vi "read_ini_SavedPos.vi"(8 "error in (no error)":errorcluster caption="错误输入（无错误）", 10 "file ref in":T1, 11 "MotorSystem 输入":refnum<class "MotorSystem.lvclass">) -> (0 "error out":errorcluster caption="错误输出", 2 "file ref out":T1, 3 "MotorSystem 输出":refnum<class "MotorSystem.lvclass">)   [LabVIEW 2016, in "MotionControl_UFO_3DOF.lvlib" / "MotorSystem.lvclass"]
uses:
  <userlib>/MotionControl_UFO_3DOF/MotorSystem/MotorSystem.lvclass
  <vilib>/Utility/config.llb/Config Data RefNum.ctl
  <userlib>/MotionControl_UFO_3DOF/MotorSystem/SavedPosCluster.ctl
  <userlib>/MotionControl_UFO_3DOF/MotorSystem/CommandList.ctl
  <userlib>/MotionControl_UFO_3DOF/MotorSystem/cmd_system.ctl
  <userlib>/MotionControl_UFO_3DOF/MotorSystem/SavedDimensionCluster.ctl
  <userlib>/MotionControl_UFO_3DOF/OneMotion/unit mode.ctl
  <userlib>/MotionControl_UFO_3DOF/MotorSystem/MotorSystem.lvclass/MotorSystem.ctl
  <vilib>/Utility/config.llb/Read Key (I32).vi
  <vilib>/Utility/config.llb/Read Key (String).vi
  <vilib>/Utility/config.llb/Read Key (Double).vi
  <vilib>/Utility/config.llb/NI_LVConfig.lvlib
  <userlib>/MotionControl_UFO_3DOF/OneMotion/OneMotion.lvclass
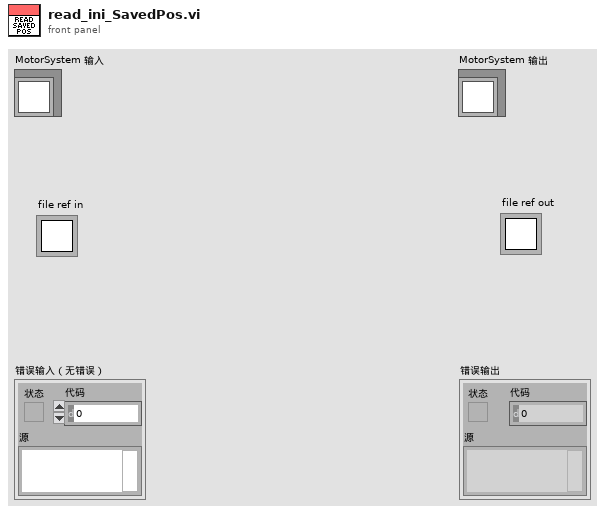
[diagram p1: front panel]
types:
  T1 = typedef "NI_LVConfig.lvlib/Config Data RefNum.ctl" = refnum<k1>
  T2 = typedef "MotionControl_UFO_3DOF.lvlib/MotorSystem.lvclass/SavedPosCluster.ctl" = cluster{"name":string, "command list":T3}
  T3 = typedef "MotionControl_UFO_3DOF.lvlib/MotorSystem.lvclass/CommandList.ctl" = cluster{"cmd":T4, "cmd info":T5[]}[]
  T4 = typedef "MotionControl_UFO_3DOF.lvlib/MotorSystem.lvclass/cmd_system.ctl" = enum16{"NONE", "MOVE_SYSTEM", "WAIT_UNTIL_MOVE_DONE", "EXIT", "WAIT_UNTIL_SELECTED_MOVE_DONE", "WAIT_A_TIME"}
  T5 = typedef "MotionControl_UFO_3DOF.lvlib/MotorSystem.lvclass/SavedDimensionCluster.ctl" = cluster{"dimension name":string, "pos":dbl, "unit mode":T6, "unit conversion ratio":dbl}
  T6 = typedef "MotionControl_UFO_3DOF.lvlib/OneMotion.lvclass/unit mode.ctl" = enum16{"motor (pulse)", "linear (mm) or radial (degree)"}
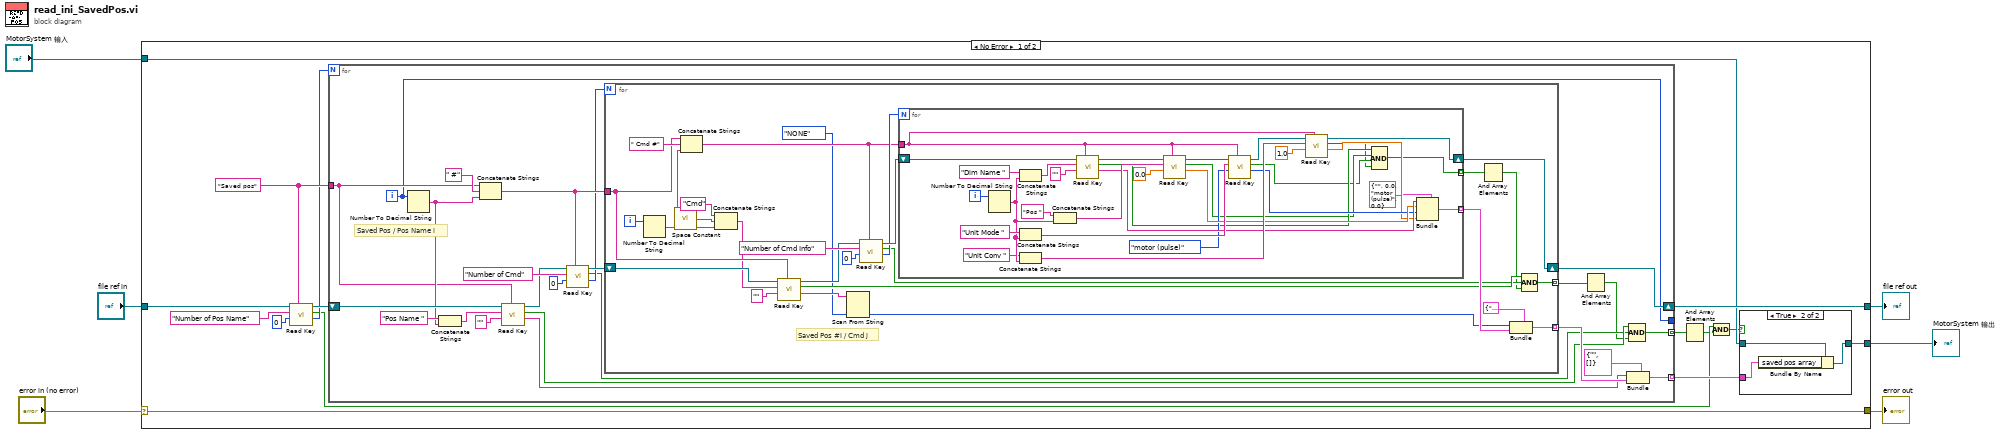
[diagram p0: block diagram]
diagram:
  n1 = case shown="No Error" "error in (no error)" {
    selector: "error in (no error)" -> [w21 w110]
    tunnel: [w21 w110] -> w5
    tunnel: [w11 w109] -> w3
    tunnel: "MotorSystem 输入" -> [w12 w109]
    tunnel: "file ref in" -> [w17 w108]
    tunnel: [w20 w108] -> w1
    frame No Error {
      w18 = "Saved pos"
      n2 = call-poly <vilib>:"Read Key.vi"("section"=w18, "default value"=0, "key"="Number of Pos Name", "refnum"=w17) -> ("value"=w14:i32, "found?"=w9:bool, "refnum out"=w16:T1)  [unwired: 4 in, 1 out]
      n3 = for {
        N: w14 -> [_]
        shift-right: [w46] -> w20
        shift-left: w16 -> [w47]
        tunnel: w18 -> [w43]
        tunnel: [w33] -> w13 mode=indexing
        tunnel: [w41] -> _
        tunnel: [w26] -> w10 mode=indexing
        i -> [w41]
        # "Saved Pos / Pos Name i"
        n4 = Number To Decimal String(number=w41) -> (decimal integer string=w44:string)  [unwired: 1 in]
        n5 = Concatenate Strings("Pos Name ", w44) -> (w48:string)
        n6 = Concatenate Strings(w43, " #", w44) -> (w39:string)
        n7 = call-poly <vilib>:"Read Key.vi"("section"=w43, "default value"="", "key"=w48, "refnum"=w47) -> ("value"=w34:string, "found?"=w29:bool, "refnum out"=w31:T1)  [unwired: 4 in, 1 out]
        n8 = call-poly <vilib>:"Read Key.vi"("section"=w39, "default value"=0, "key"="Number of Cmd", "refnum"=w31) -> ("value"=w36:i32, "found?"=w28:bool, "refnum out"=w38:T1)  [unwired: 4 in, 1 out]
        n9 = for {
          N: w36 -> [_]
          tunnel: w39 -> [w69]
          tunnel: [w61] -> w35 mode=indexing
          shift-right: [w76] -> w46
          shift-left: w38 -> [w73]
          tunnel: [w54] -> w30 mode=indexing
          i -> [w70]
          # "Saved Pos #i / Cmd j"
          n10 = Number To Decimal String(number=w70) -> (decimal integer string=w72:string)  [unwired: 1 in]
          n11 = call <vilib>:"Space Constant.vi"() -> ("String"=w68:string)
          n12 = Concatenate Strings(w69, " Cmd #", w72) -> (w63:string)
          n13 = Concatenate Strings("Cmd", w68, w72) -> (w67:string)
          n14 = call-poly <vilib>:"Read Key.vi"("section"=w69, "default value"="", "key"=w67, "refnum"=w73) -> ("value"=w53:string, "found?"=w57:bool, "refnum out"=w58:T1)  [unwired: 4 in, 1 out]
          n15 = Scan From String(input string=w53, default 1=cmd_system."NONE" ("cmd")) -> (output 1=w50:T4)  [unwired: 3 in, 3 out]
          n16 = call-poly <vilib>:"Read Key.vi"("section"=w63, "default value"=0, "key"="Number of Cmd Info", "refnum"=w58) -> ("value"=w64:i32, "found?"=w56:bool, "refnum out"=w65:T1)  [unwired: 4 in, 1 out]
          n17 = for {
            N: w64 -> [_]
            shift-right: [w95] -> w76
            shift-left: w65 -> [w106]
            tunnel: w63 -> [w94]
            tunnel: [w85] -> w62 mode=indexing
            tunnel: [w77] -> w59 mode=indexing
            i -> [w84]
            n18 = Number To Decimal String(number=w84) -> (decimal integer string=w101:string)  [unwired: 1 in]
            n19 = Concatenate Strings("Dim Name ", w101) -> (w93:string)
            n20 = Concatenate Strings("Unit Mode ", w101) -> (w98:string)
            n21 = Concatenate Strings("Unit Conv ", w101) -> (w99:string)
            n22 = Concatenate Strings("Pos ", w101) -> (w104:string)
            n23 = call-poly <vilib>:"Read Key.vi"("section"=w94, "default value"="", "key"=w93, "refnum"=w106) -> ("value"=w91:string, "found?"=w81:bool, "refnum out"=w103:T1)  [unwired: 4 in, 1 out]
            n24 = call-poly <vilib>:"Read Key.vi"("section"=w94, "default value"=0.0, "key"=w104, "refnum"=w103) -> ("value"=w89:dbl, "found?"=w80:bool, "refnum out"=w97:T1)  [unwired: 4 in, 1 out]
            n25 = call-poly <vilib>:"Read Key.vi"("section"=w94, "default value"=unit_mode."motor (pulse)" ("unit mode"), "key"=w98, "refnum"=w97) -> ("value"=w87:i32, "found?"=w79:bool, "refnum out"=w96:T1)  [unwired: 4 in, 1 out]
            n26 = call-poly <vilib>:"Read Key.vi"("section"=w94, "default value"=1.0, "key"=w99, "refnum"=w96) -> ("value"=w86:dbl, "found?"=w78:bool, "refnum out"=w95:T1)  [unwired: 4 in, 1 out]
            n27 = Compound Arithmetic op=AND(w81, w80, w79, w78) -> (w77:bool)
            n28 = Bundle(cluster=T5 {"dimension name"="", "pos"=0.0, "unit mode"=enum."motor (pulse)", "unit conversion ratio"=0.0} ("a dimension cluster"), "dimension name"=w91, "pos"=w89, "unit mode"=w87, "unit conversion ratio"=w86) -> (w85:T5)
          }
          n29 = And Array Elements(Boolean array=w59) -> (logical AND=w55:bool)
          n30 = Bundle(cluster=cluster{"cmd":T4, "cmd info":T5[]} {"cmd"=enum."NONE", "cmd info"=[]} ("a saved pos"), "cmd"=w50, "cmd info"=w62) -> (w61:cluster{"cmd":T4, "cmd info":T5[]})
          n31 = Compound Arithmetic op=AND(w57, w56, w55) -> (w54:bool)
        }
        n32 = And Array Elements(Boolean array=w30) -> (logical AND=w27:bool)
        n33 = Bundle(cluster=T2 {"name"="", "command list"=[]} ("a saved pos cluster"), "name"=w34, "command list"=w35) -> (w33:T2)
        n34 = Compound Arithmetic op=AND(w29, w28, w27) -> (w26:bool)
      }
      n35 = And Array Elements(Boolean array=w10) -> (logical AND=w8:bool)
      n36 = Compound Arithmetic op=AND(w9, w8) -> (w7:bool)
      n37 = case shown="True" w7 {
        tunnel: w13 -> [_ w25]
        tunnel: w12 -> [w22 w24]
        tunnel: [w22 w23] -> w11
        frame False {
        }
        frame True {
          n38 = Bundle By Name(cluster=w24, "saved pos array"=w25) -> (w23:refnum<class "MotorSystem.lvclass">)
        }
      }
    }
    frame Error {
    }
  }
  "error out" <- w5
  "MotorSystem 输出" <- w3
  "file ref out" <- w1
